vi "SSH Set .NET Refnum.vi"(8 "Error In":errorcluster, 10 "SSH .NET Refnum":refnum<k24>, 11 "SSH Session":refnum<k1>) -> (0 "Error Out":errorcluster, 3 "SSH Session":refnum<k1>)   [LabVIEW 2020, in "LMH-LINX.lvlib"]
uses:
  LMH-LINX.lvlib
  c:/p4/penguin/lvaddon/MakerHub/LINX/trunk/20.1/objects/MakerHub_LINX/win32U/i386/msvc90/release/LabVIEW/vi.lib/MakerHub/LINX/Resources/Renci.SshNet.dll
  Resources/Renci.SshNet.dll
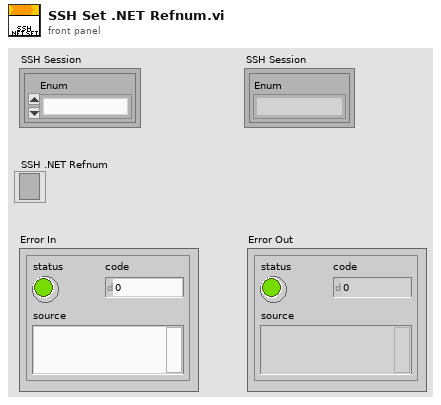
[diagram p1: front panel]
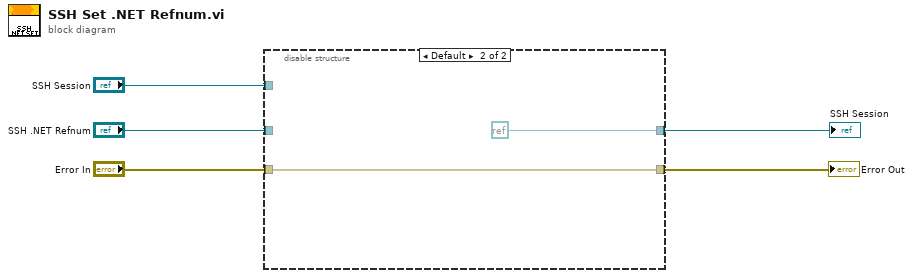
[diagram p0: block diagram]
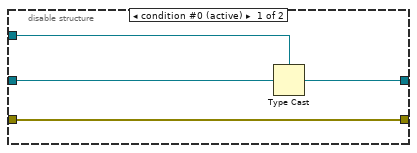
[diagram p2: hidden frame]
diagram:
  n1 = disable-structure shown="Default" {
    disable-tunnel: [w9 w11] -> w4
    disable-tunnel: "Error In" -> [w9 w11]
    disable-tunnel: "SSH Session" -> [w6 _]
    disable-tunnel: [w8 refnum<k0> refnum] -> w1
    disable-tunnel: "SSH .NET Refnum" -> [w7 _]
    frame condition #0 (active) {
      n2 = Type Cast(type=w6, x=w7) -> (*(type *) &x=w8:refnum<k1>)
    }
    frame condition #1 {
    }
  }
  "Error Out" <- w4
  "SSH Session" <- w1
